vi "decimateAllMatrix_singleAxis.vi"(10 "AllMatrix":dbl[](array[numeric]), 11 "NS_obs/cntrl":u8) -> (2 "ControlMatrices":T1, 4 "remaining_array":dbl[](array[numeric]))   [LabVIEW 2017]
uses:
  ObserverMatrices.ctl
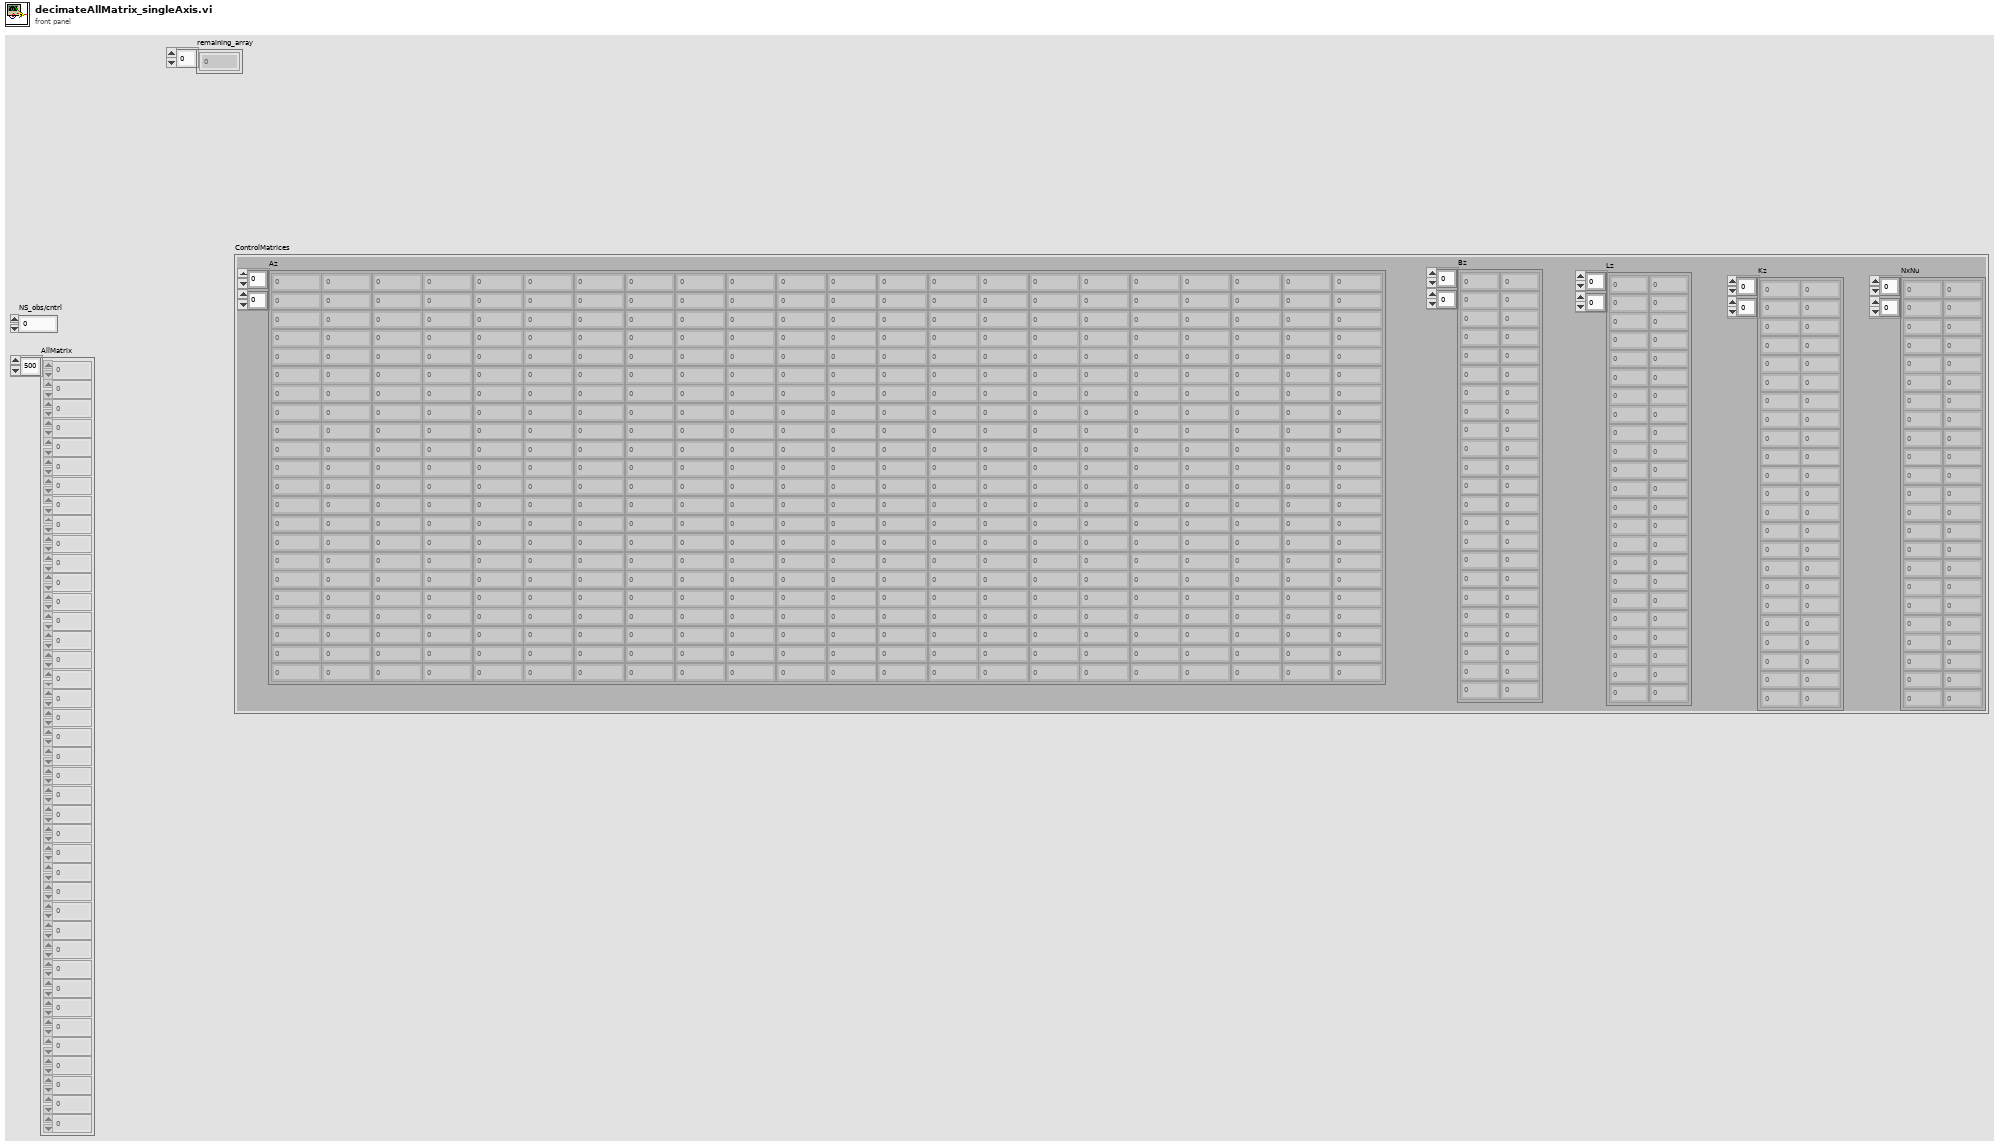
[diagram p1: front panel]
types:
  T1 = typedef "ObserverMatrices.ctl" = cluster{"Az":fxp<+/-,32,4>[][], "Bz":dbl[][], "Lz":dbl[][], "Kz":dbl[][], "NxNu":dbl[][]}
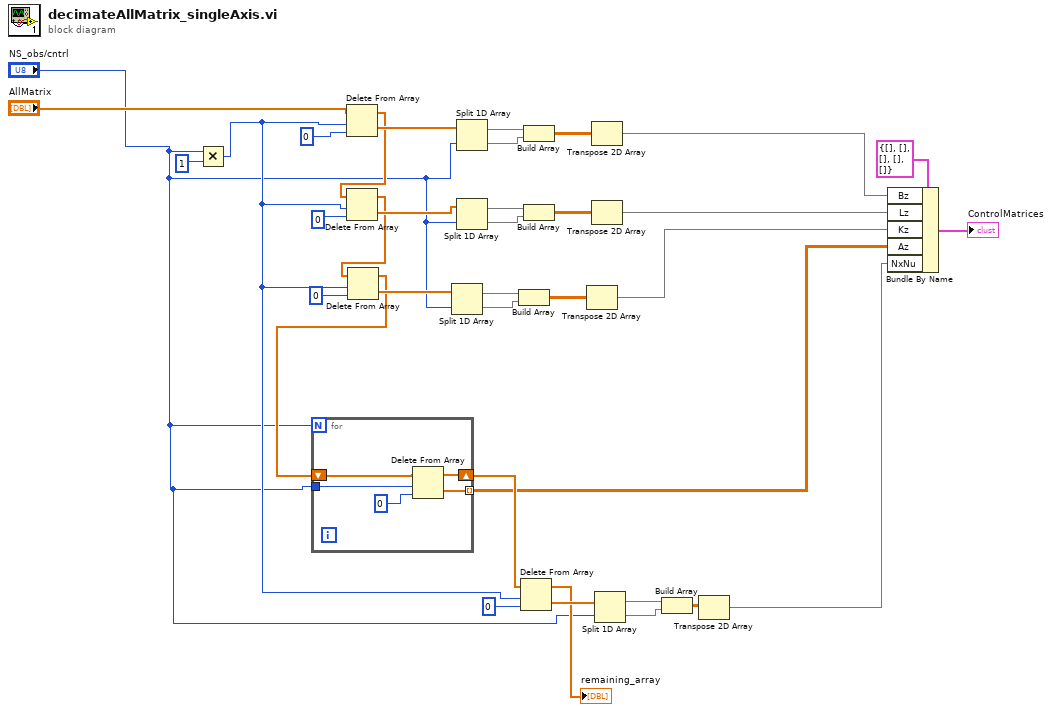
[diagram p0: block diagram]
diagram:
  n1 = Multiply(x="NS_obs/cntrl", y=u8 1) -> (x*y=w20:u8)
  n2 = Delete From Array(array="AllMatrix", length=w20, index=0) -> (deleted portion=w23:dbl[], array with subset deleted=w12:dbl[])
  n3 = Delete From Array(array=w12, length=w20, index=0) -> (deleted portion=w28:dbl[], array with subset deleted=w14:dbl[])
  n4 = Delete From Array(array=w14, length=w20, index=0) -> (deleted portion=w32:dbl[], array with subset deleted=w19:dbl[])
  n5 = for {
    N: "NS_obs/cntrl" -> [_]
    shift-right: [w37] -> w17
    shift-left: w19 -> [w40]
    tunnel: "NS_obs/cntrl" -> [w39]
    tunnel: [w38] -> w6 mode=indexing
    n6 = Delete From Array(array=w40, length=w39, index=0) -> (deleted portion=w38:dbl[], array with subset deleted=w37:dbl[])
  }
  n7 = Split 1D Array(array=w32, index="NS_obs/cntrl") -> (first subarray=w29:dbl[], second subarray=w30:dbl[])
  n8 = Split 1D Array(array=w23, index="NS_obs/cntrl") -> (first subarray=w21:dbl[], second subarray=w22:dbl[])
  n9 = Split 1D Array(array=w28, index="NS_obs/cntrl") -> (first subarray=w25:dbl[], second subarray=w26:dbl[])
  n10 = Build Array(w29, w30) -> (w31:dbl[][])
  n11 = Delete From Array(array=w17, length=w20, index=0) -> (deleted portion=w36:dbl[], array with subset deleted=→"remaining_array":dbl[])
  n12 = Build Array(w21, w22) -> (w24:dbl[][])
  n13 = Build Array(w25, w26) -> (w27:dbl[][])
  n14 = Transpose 2D Array(2D array=w31) -> (transposed array=w8:dbl[][])
  n15 = Transpose 2D Array(2D array=w24) -> (transposed array=w10:dbl[][])
  n16 = Transpose 2D Array(2D array=w27) -> (transposed array=w9:dbl[][])
  n17 = Split 1D Array(array=w36, index="NS_obs/cntrl") -> (first subarray=w33:dbl[], second subarray=w34:dbl[])
  n18 = Build Array(w33, w34) -> (w35:dbl[][])
  n19 = Transpose 2D Array(2D array=w35) -> (transposed array=w5:dbl[][])
  n20 = Bundle By Name(cluster=T1 {"Az"=[], "Bz"=[], "Lz"=[], "Kz"=[], "NxNu"=[]} ("ControlMatrices 2"), "Bz"=w10, "Lz"=w9, "Kz"=w8, "Az"=w6, "NxNu"=w5) -> (→"ControlMatrices":T1)
